vi "FPGA_SystemOpen.vi"() -> (0 "error out":errorcluster, 3 "FRC FPGA Ref":T1)   [LabVIEW 2017]
uses:
  <vilib>/Rock Robotics/SystemInterfaces/System/FPGA_SystemFRC FPGA Ref.ctl
  <vilib>/Utility/error.llb/Error Cluster From Error Code.vi
  <vilib>/rvi/errors/niLvFpgaAdjustHostInterfaceError.vi
  <vilib>/rvi/interface/nirviReadWriteControl/nirviReadWriteControl.xnode
  <vilib>/rvi/interface/nirviOpenFPGA/nirviOpenFPGA.xnode
  NiFpgaLv.dll
  <vilib>/rvi/interface/Simulation/niFpgaSimulationCallBeginRW.vi
  <vilib>/Rock Robotics/SystemInterfaces/roboRIO_FPGA_2018_18.0.8.lvbitx
  <vilib>/FPGAPlugInAG/roboRIO/niLvFpga_Open_roboRIO.vi
  <vilib>/rvi/interface/common/dynamic/niFpgaDynamicAddResources.vi
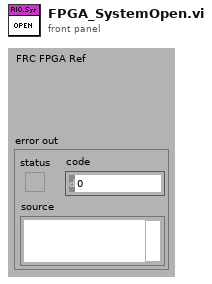
[diagram p1: front panel]
types:
  T1 = typedef "FPGA_SystemFRC FPGA Ref.ctl" = refnum<k20>
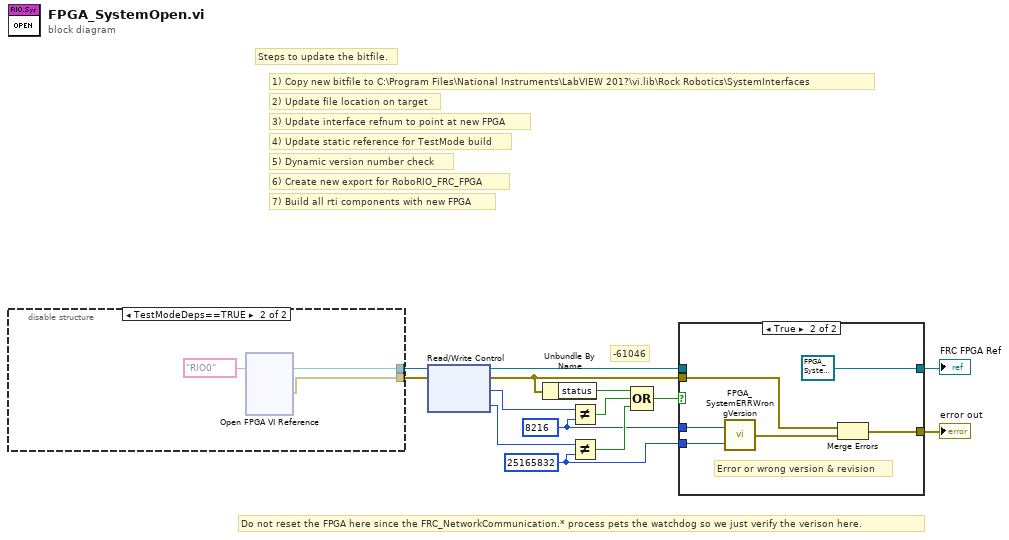
[diagram p0: block diagram]
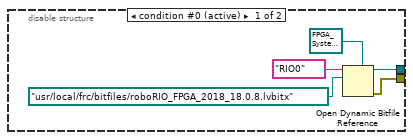
[diagram p2: hidden frame]
diagram:
  w3 = u32 25165832
  w4 = u16 8216
  # "3) Update interface refnum to point at new FPGA"
  # "7) Build all rti components with new FPGA"
  # "6) Create new export for RoboRIO_FRC_FPGA"
  # "1) Copy new bitfile to C:\\Program Files\\National Instruments\\LabVIEW 201?\\vi.lib\\Rock Robotics\\SystemInterfaces"
  # "5) Dynamic version number check"
  # "4) Update static reference for TestMode build"
  # "Steps to update the bitfile."
  # "2) Update file location on target"
  # "-61046"
  # "Do not reset the FPGA here since the FRC_NetworkCommunication.* process pets the watchdog so we just verify the verison here."
  n1 = disable-structure shown="TestModeDeps==TRUE" {
    disable-tunnel: [w15 w21] -> w2
    disable-tunnel: [w16 w20] -> w1
    frame condition #0 (active) {
      n2 = Open Dynamic Bitfile Reference(0:tag "RIO0" ("resource name"), 1:path "/usr/local/frc/bitfiles/roboRIO_FPGA_2018_18.0.8.lvbitx" ("Bitfile path"), 4:T1 refnum ("FRC FPGA Ref")) -> (5:w16:T1, 8:w15:errorcluster)  [unwired: 2 in]
    }
    frame condition #1 {
      n3 = xnode "Open FPGA VI Reference"("resource name"=tag "RIO0") -> ("FPGA VI Reference Out"=w20:refnum<k20>, "error out"=w21:errorcluster)  [unwired: 1 in]
    }
  }
  n4 = xnode "Read/Write Control"("FPGA VI Reference In"=w1, "error in"=w2) -> ("FPGA VI Reference Out"=w12:T1, "error out"=w10:errorcluster, "Version"=w8:u16, "Revision"=w7:u32)
  n5 = Unbundle By Name(w10) -> ("status"=w11:bool)
  n6 = Not Equal?(x=w8, y=w4) -> (x != y?=w6:bool)
  n7 = Not Equal?(x=w7, y=w3) -> (x != y?=w5:bool)
  n8 = Compound Arithmetic op=OR(w11, w6, w5) -> (w9:bool)
  n9 = case shown="True" w9 {
    tunnel: [w24 T1 refnum ("FRC FPGA Ref")] -> w14
    tunnel: w12 -> [w24 _]
    tunnel: [w23 w25] -> w13
    tunnel: w10 -> [w23 w27]
    tunnel: w4 -> [_ w29]
    tunnel: w3 -> [_ w28]
    frame False {
    }
    frame True {
      # "Error or wrong version & revision"
      n10 = call <vilib>:"FPGA_SystemERRWrongVersion.vi"("Revision"=w28, "Version"=w29) -> ("error out"=w26:errorcluster)  [unwired: 1 out]
      n11 = Merge Errors(w27, w26) -> (w25:errorcluster)
    }
  }
  "error out" <- w13
  "FRC FPGA Ref" <- w14
